vi "cube plot.vi"() -> ()   [LabVIEW 2020]
panel:
  in  "Numeric":i32=50
  out "Waveform Graph":i32[][](graph)
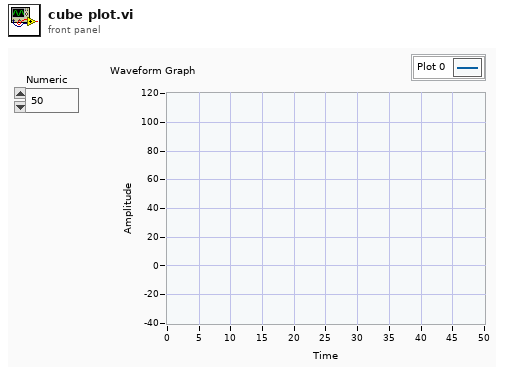
[diagram p1: front panel]
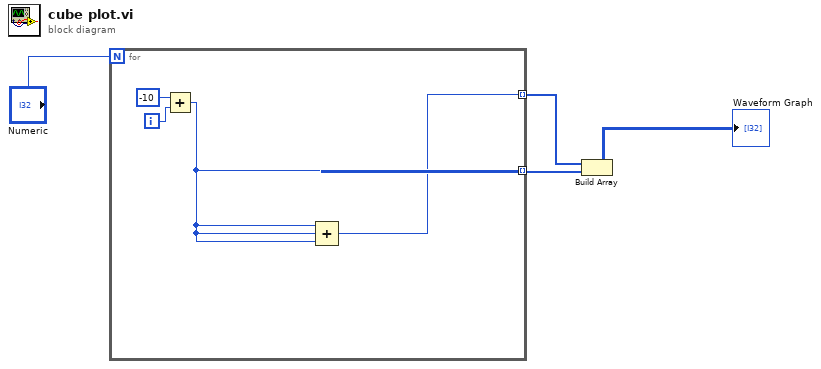
[diagram p0: block diagram]
diagram:
  n1 = for {
    N: "Numeric" -> [_]
    tunnel: [w6] -> w4 mode=indexing
    tunnel: [w5] -> w3 mode=indexing
    i -> [w8]
    n2 = Add(x=-10, y=w8) -> (x+y=w6:i32)
    n3 = Compound Arithmetic op=ADD(w6, w6, w6) -> (w5:i32)
  }
  n4 = Build Array "Build Array"(w3, w4) -> (→"Waveform Graph":i32[][])
